vi "etapa_2.vi"() -> ()   [LabVIEW 2017]
uses:
  <vilib>/Analysis/2dsp.llb/Real FFT.vi
  <vilib>/LabVIEW Interface for Arduino/LabVIEW Interface for Arduino.lvlib
  <vilib>/Analysis/NI_AALPro.lvlib
panel:
  in  "N Amostras":u16
  out "FFT":dbl[](graph) caption="Waveform Chart"
  in  "stop":bool
  in  "Sample rate (Hz)":u16
  in  "Analog input pin":u8
  out "error out":errorcluster
  in  "VISA resource":refnum<visa-resource-name>
  out "Waveform Chart":dbl[](graph)
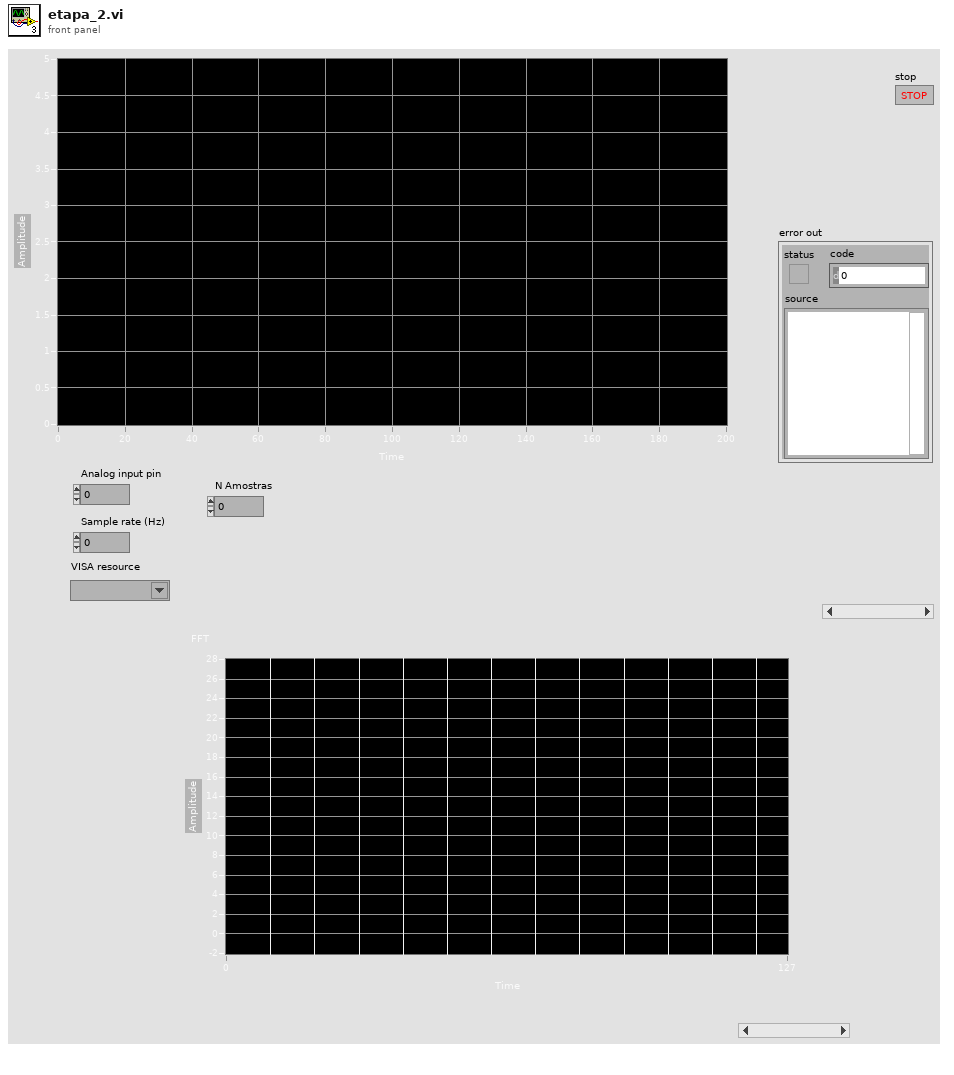
[diagram p1: front panel]
types:
  T1 = typedef "LabVIEW Interface for Arduino.lvlib/Arduino Resource.ctl" = cluster{"VISA resource":refnum<visa-resource-name>, "Board Type":T2, "Connection Type":enum8{"USB / Serial"}, "Bytes Per Packet (15)":u8}
  T2 = typedef "LabVIEW Interface for Arduino.lvlib/Board Type.ctl" = enum16{"Uno", "Dimuelanove w/Atmega 328", "Mega 2560"}
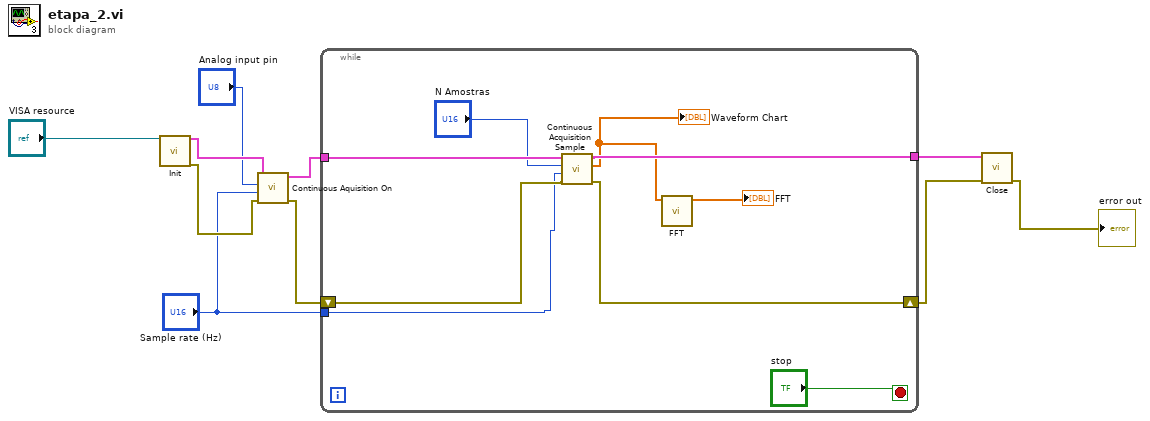
[diagram p0: block diagram]
diagram:
  n1 = call <vilib>:"Init.vi"("VISA resource"="VISA resource") -> ("Arduino Resource"=w9:T1, "error out"=w7:errorcluster)  [unwired: 17 in]
  n2 = call <vilib>:"Continuous Aquisition On.vi"("error in"=w7, "Acquition Speed"="Sample rate (Hz)", "Analog Input Pin"="Analog input pin", "Arduino Resource"=w9) -> ("error out"=w6:errorcluster, "Arduino Resource"=w8:T1)  [unwired: 6 in]
  n3 = while {
    tunnel: w8 -> [w18]
    tunnel: "Sample rate (Hz)" -> [w12]
    tunnel: [w17] -> w3
    shift-right: [w16] -> w2
    shift-left: w6 -> [w15]
    stop <- "stop" stop-if-true
    n4 = call <vilib>:"Continuous Acquisition Sample.vi"("Arduino Resource"=w18, "Samples to Read"="N Amostras", "Sample Rate (HZ)"=w12, "error in (no error)"=w15) -> ("Arduino Resource"=w17:T1, "Data"=w14:dbl[], "error out"=w16:errorcluster)  [unwired: 4 in]
    "Waveform Chart" <- w14
    n5 = call-poly <vilib>:"FFT.vi"("X"=w14) -> ("FFT {X}"=→"FFT":cdb[])  [unwired: 9 in, 1 out]
  }
  n6 = call <vilib>:"Close.vi"("Arduino Resource"=w3, "error in"=w2) -> ("error out"=→"error out":errorcluster)  [unwired: 13 in]
